vi "Front Panel Cleanup.vi"(8 "error in":errorcluster, 11 "vi refnum":refnum<vi>) -> (0 "error out":errorcluster, 3 "vi refnum out":refnum<vi>)   [LabVIEW 2021, in "MeasurementClient Editor.lvlib"]
uses:
  MeasurementClient Editor.lvlib
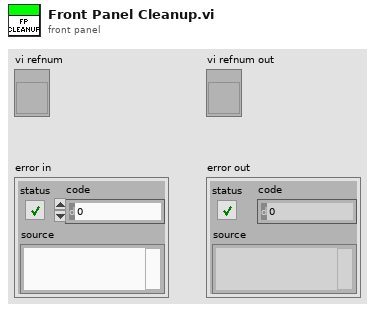
[diagram p1: front panel]
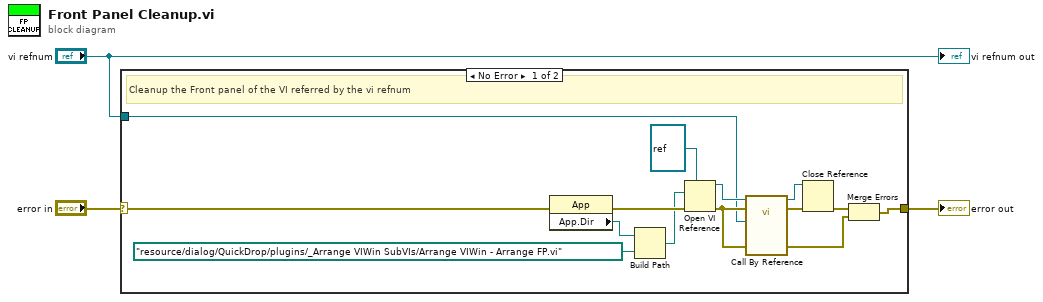
[diagram p0: block diagram]
diagram:
  n1 = case shown="No Error" "error in" {
    selector: "error in" -> [w17 w18]
    tunnel: [w12 w18] -> w3
    tunnel: "vi refnum" -> [w4 _]
    frame No Error {
      # "Cleanup the Front panel of the VI referred by the vi refnum"
      n2 = property class="App"(error in=w17) -> (error out=w16:errorcluster, "App.Dir"=w15:path)  [unwired: 1 in, 1 out]
      n3 = Build Path(base path=w15, name or relative path=path "resource/dialog/QuickDrop/plugins/_Arrange VIWin SubVIs/Arrange VIWin - Arrange FP.vi") -> (appended path=w10:path)
      n4 = Open VI Reference(type specifier VI Refnum (for type only)=refnum<vi> refnum, vi path=w10, error in (no error)=w16) -> (vi reference=w8:refnum<vi>, error out=w5:errorcluster)  [unwired: 3 in]
      n5 = call-by-ref "?"(reference=w8, error in=w5, "VI"=w4, "error in"=w5) -> (reference out=w7:refnum<vi>, error out=w9:errorcluster, 15:"error out"=w6:errorcluster)  [unwired: 13 in]
      n6 = Close Reference(reference=w7, error in (no error)=w9) -> (error out=w11:errorcluster)
      n7 = Merge Errors(w11, w6) -> (w12:errorcluster)
    }
    frame Error {
      # "Pass"
    }
  }
  "error out" <- w3
  "vi refnum out" <- "vi refnum"
